vi "Get_command.vi"() -> ()   [LabVIEW 2020]
uses:
  VNA-Commands.ctl
  VNA-Addresses.ctl
panel:
  out "Address":u16 format="%x"
  out "Command":u16 format="%x"
  out "CMDADDR":u32 format="%x"
  in  "Address":T1
  in  "Commands":T2
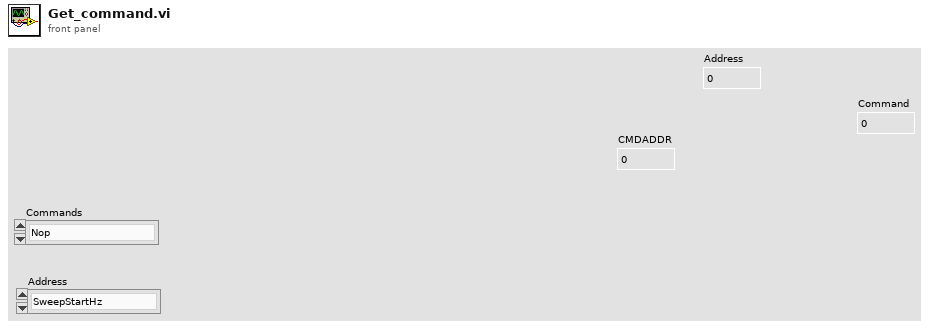
[diagram p1: front panel]
types:
  T1 = typedef "VNA-Addresses.ctl" = enum16{"SweepStartHz", "SweepStopHz", "SweepPoints", "valuesPerFrequency", "RawSamplesMode", "ValuesFIFO", "deviceVariant", "protocolVersion", "hardwareRevision", "firmwareMajor", ""}
  T2 = typedef "VNA-Commands.ctl" = enum16{"Nop", "Indicate", "Read 1B", "Read 2B", "Read 4B", "Read 8B", "Read FIFO", "Write 1B", "Write 2B", "Write 4B", "Write 8B", "Write FIFO"}
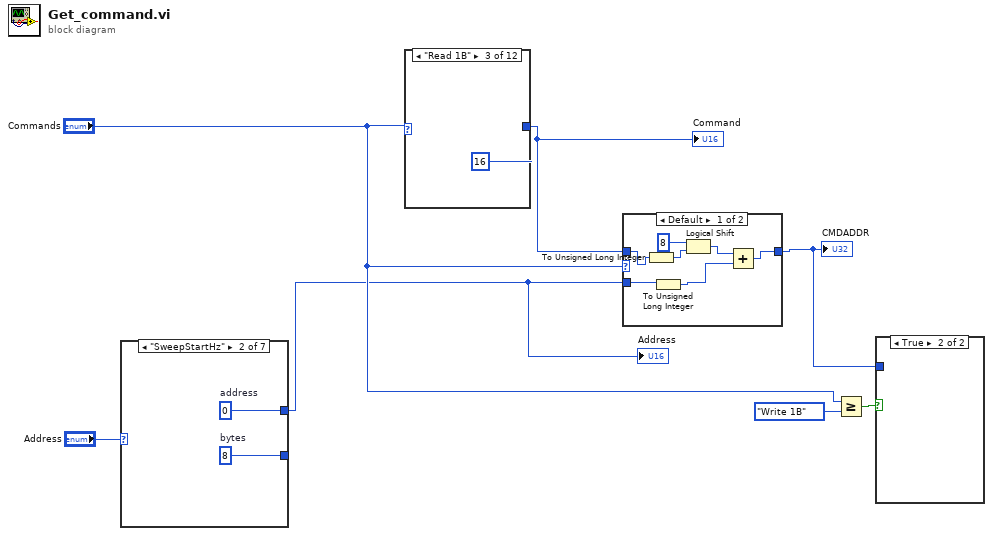
[diagram p0: block diagram]
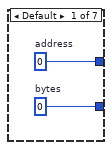
[diagram p2: hidden frame]
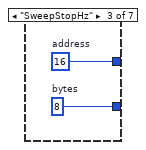
[diagram p3: hidden frame]
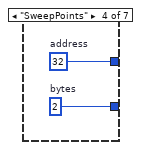
[diagram p4: hidden frame]
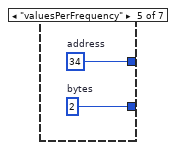
[diagram p5: hidden frame]
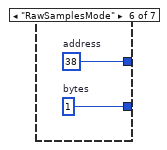
[diagram p6: hidden frame]
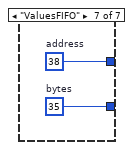
[diagram p7: hidden frame]
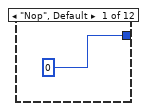
[diagram p9: hidden frame]
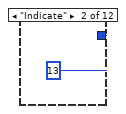
[diagram p10: hidden frame]
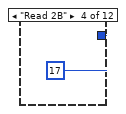
[diagram p11: hidden frame]
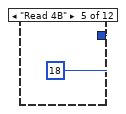
[diagram p12: hidden frame]
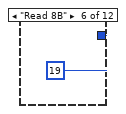
[diagram p13: hidden frame]
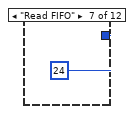
[diagram p14: hidden frame]
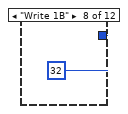
[diagram p15: hidden frame]
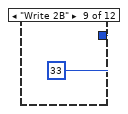
[diagram p16: hidden frame]
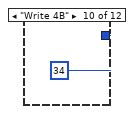
[diagram p17: hidden frame]
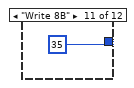
[diagram p18: hidden frame]
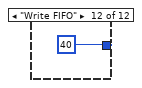
[diagram p19: hidden frame]
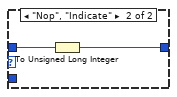
[diagram p20: hidden frame]
diagram:
  n1 = case shown="\"SweepStartHz\"" "Address" {
    tunnel: [w9 w11 w13 w15 w17 w19 w21] -> w2
    tunnel: [w8 w10 w12 w14 w16 w18 w20] -> _
    frame Default {
      w8 = 0  # bytes
      w9 = u16 0  # address
    }
    frame "SweepStartHz" {
      w10 = 8  # bytes
      w11 = u16 0  # address
    }
    frame "SweepStopHz" {
      w12 = 8  # bytes
      w13 = u16 16  # address
    }
    frame "SweepPoints" {
      w14 = 2  # bytes
      w15 = u16 32  # address
    }
    frame "valuesPerFrequency" {
      w16 = 2  # bytes
      w17 = u16 34  # address
    }
    frame "RawSamplesMode" {
      w18 = 1  # bytes
      w19 = u16 38  # address
    }
    frame "ValuesFIFO" {
      w20 = 35  # bytes
      w21 = u16 38  # address
    }
  }
  "Address" <- w2
  n2 = case shown="\"Read 1B\"" "Commands" {
    tunnel: [u16 0 u16 13 u16 16 u16 17 u16 18 u16 19 u16 24 u16 32 u16 33 u16 34 u16 35 u16 40] -> w3
    frame "Nop", Default {
    }
    frame "Indicate" {
    }
    frame "Read 1B" {
    }
    frame "Read 2B" {
    }
    frame "Read 4B" {
    }
    frame "Read 8B" {
    }
    frame "Read FIFO" {
    }
    frame "Write 1B" {
    }
    frame "Write 2B" {
    }
    frame "Write 4B" {
    }
    frame "Write 8B" {
    }
    frame "Write FIFO" {
    }
  }
  "Command" <- w3
  n3 = case shown="Default" "Commands" {
    tunnel: w3 -> [w38 w42]
    tunnel: w2 -> [w35 _]
    tunnel: [w36 w41] -> w1
    frame Default {
      n4 = To Unsigned Long Integer(number=w38) -> (unsigned 32bit integer=w39:u32)
      n5 = To Unsigned Long Integer(number=w35) -> (unsigned 32bit integer=w34:u32)
      n6 = Logical Shift(y=i16 8, x=w39) -> (x << y=w37:u32)
      n7 = Add(x=w37, y=w34) -> (x+y=w36:u32)
    }
    frame "Nop", "Indicate" {
      n8 = To Unsigned Long Integer(number=w42) -> (unsigned 32bit integer=w41:u32)
    }
  }
  "CMDADDR" <- w1
  n9 = Greater Or Equal?(x="Commands", y=VNA-Commands."Write 1B") -> (x >= y?=w5:bool)
  n10 = case shown="True" w5 {
    tunnel: w1 -> [_ _]
    frame False {
    }
    frame True {
    }
  }
